vi "OtherGoalsCrosshair.vi"(9 "FullArray":dbl[][](array[numeric]), 10 "SelectedGoalSubarray":dbl[](array[numeric]), 11 "Image In":T1) -> (3 "Image Out":T1)   [LabVIEW 2012]
uses:
  <vilib>/vision/Image Controls.llb/IMAQ Image.ctl
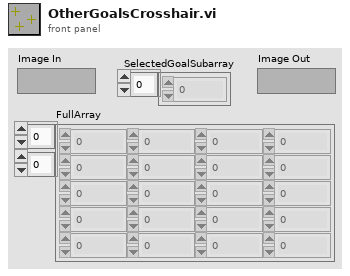
[diagram p1: front panel]
types:
  T1 = typedef "IMAQ Image.ctl" = refnum<image>
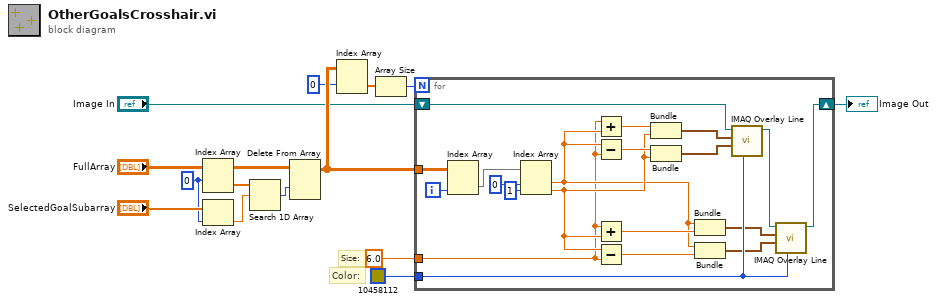
[diagram p0: block diagram]
diagram:
  w7 = 0 ("index (row)")
  # "Color:"
  # "Size:"
  n1 = Index Array(array="FullArray", index (row)=w7) -> (element=w14:dbl[])  [unwired: 1 in]
  n2 = Index Array(array="SelectedGoalSubarray", index=w7) -> (element=w9:dbl)
  n3 = Search 1D Array(1D array=w14, element=w9) -> (index of element=w13:i32)  [unwired: 1 in]
  n4 = Delete From Array(array="FullArray", index (row)=w13) -> (array with subset deleted=w6:dbl[][])  [unwired: 2 in, 1 out]
  n5 = Index Array(array=w6, index (row)=0) -> (element=w11:dbl[])  [unwired: 1 in]
  n6 = Array Size(array=w11) -> (size(s)=w5:i32)
  n7 = for {
    N: w5 -> [_]
    tunnel: w6 -> [w19]
    tunnel: 6.0 ("x") -> [w16]
    tunnel: u32 10458112 ("Color") -> [w34]
    shift-right: [w20] -> w8
    shift-left: "Image In" -> [w15]
    i -> [w17]
    n8 = Index Array(array=w19, index (col)=w17) -> (element=w18:dbl[])  [unwired: 1 in]
    n9 = Index Array(array=w18, index #1=0 ("index"), index #2=1 ("index")) -> (element #1=w21:dbl, element #2=w29:dbl)
    n10 = Add(x=w16, y=w21) -> (x+y=w30:dbl)
    n11 = Subtract(x=w21, y=w16) -> (x-y=w31:dbl)
    n12 = Add(x=w16, y=w29) -> (x+y=w24:dbl)
    n13 = Subtract(x=w29, y=w16) -> (x-y=w23:dbl)
    n14 = Bundle(w30, "Numeric"=w29) -> (w28:cluster{dbl, "Numeric":dbl})  [unwired: 1 in]
    n15 = Bundle(w31, "Numeric"=w29) -> (w27:cluster{dbl, "Numeric":dbl})  [unwired: 1 in]
    n16 = Bundle("Numeric"=w21, w24) -> (w26:cluster{"Numeric":dbl, dbl})  [unwired: 1 in]
    n17 = Bundle("Numeric"=w21, w23) -> (w25:cluster{"Numeric":dbl, dbl})  [unwired: 1 in]
    n18 = call "IMAQ Overlay Line"("Color"=w34, "End Point"=w27, "Start Point"=w28, "Image"=w15) -> ("Image Out"=w22:T1)  [unwired: 6 in, 1 out]
    n19 = call "IMAQ Overlay Line"("Color"=w34, "End Point"=w25, "Start Point"=w26, "Image"=w22) -> ("Image Out"=w20:T1)  [unwired: 6 in, 1 out]
  }
  "Image Out" <- w8
